vi "init_channel.vi"(8 "error in (no error)":errorcluster, 9 "spectrum channel type (stiched)":T1=enum."STICHED", 10 "channel DUT (index)":i32, 11 "Thorlabs_OSA200_64 in":refnum<class "OSA200.lvclass">) -> (0 "error out":errorcluster, 3 "Thorlabs_OSA200_64 out":refnum<class "OSA200.lvclass">)   [LabVIEW 2010, in "OSA200.lvclass"]
doc: "OSA200 use one channel, (OSA300 supports multichannel configurations)."
uses:
  OSA200.lvclass
  OSA.lvclass
  typeDef/channelType_spectrum.ctl
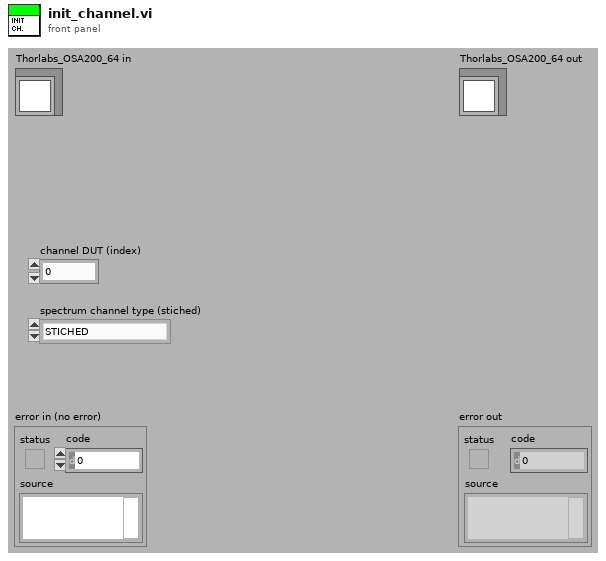
[diagram p1: front panel]
types:
  T1 = typedef "OSA.lvclass/channelType_spectrum.ctl" = enum16{"SINGLE CHANNEL", "STICHED"}
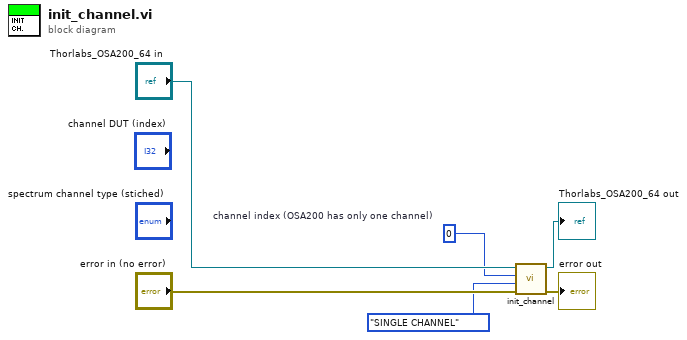
[diagram p0: block diagram]
diagram:
  w2 = 0  # channel index (OSA200 has only one channel)
  n1 = call-parent "init_channel.vi"("error in (no error)"="error in (no error)", 9:channelType_spectrum."SINGLE CHANNEL" ("spectrum channel type"), "channel index"=w2, "Thorlabs_OSA_64 in"="Thorlabs_OSA200_64 in") -> ("error out"=→"error out":errorcluster, "Thorlabs_OSA_64 out"=→"Thorlabs_OSA200_64 out":refnum<class "OSA200.lvclass">)  [unwired: 6 in]
